vi "Main_scan.vi"() -> ()   [LabVIEW 2018]
uses:
  Positional stage/G/Control 1.ctl
  D:/Labview/examples/Instrument IO/Serial/support/Serial - Settings.ctl
  D:/Labview/examples/Instrument IO/Serial/support/Serial - XON-XOFF Characters.ctl
  D:/Labview/examples/Instrument IO/Serial/support/Serial - ASCII Characters.ctl
  <vilib>/Instr/_visa.llb/VISA Configure Serial Port (Instr).vi
  <vilib>/Utility/file.llb/Write Delimited Spreadsheet (DBL).vi
panel:
  in  "Saves per point":i32
  out "Pixel Number":dbl[](array[numeric])
  out "Wavelength":dbl[](array[numeric])
  in  "St":refnum<visa-resource-name>="COM1"
  in  "Averages":u32=1 min=1 max=60000 step=1
  in  "Integration Time":u32=50 min=50 max=60000 step=1
  out "Waveform Graph 2":dbl[](graph)
  out "I num":i32
  in  "Translation Stage":refnum<visa-resource-name>="COM1"
  out "Translation Error":bool=TRUE
  out "TS Error":bool
  in  "Filenumber":u32=1
  in  "Y Interval":dbl
  in  "X Interval":dbl
  in  "Y Scan Number":dbl
  in  "X Scan Number":dbl
  in  "Scan":bool
  out "Position":string
  in  "Command":string="0x 0y"
  in  "Connect":bool=TRUE
  in  "Move":bool
  in  "Current Position":string
  out "Array":dbl[](array[numeric])
  in  "HeadFolder":T1=path "C:/Users/xinghua/Desktop/try_step"
  out "Image array":dbl[][](array[numeric])
  # "Average"
  # "Intergration time"
  # "Spec port"
  # "Single Move"
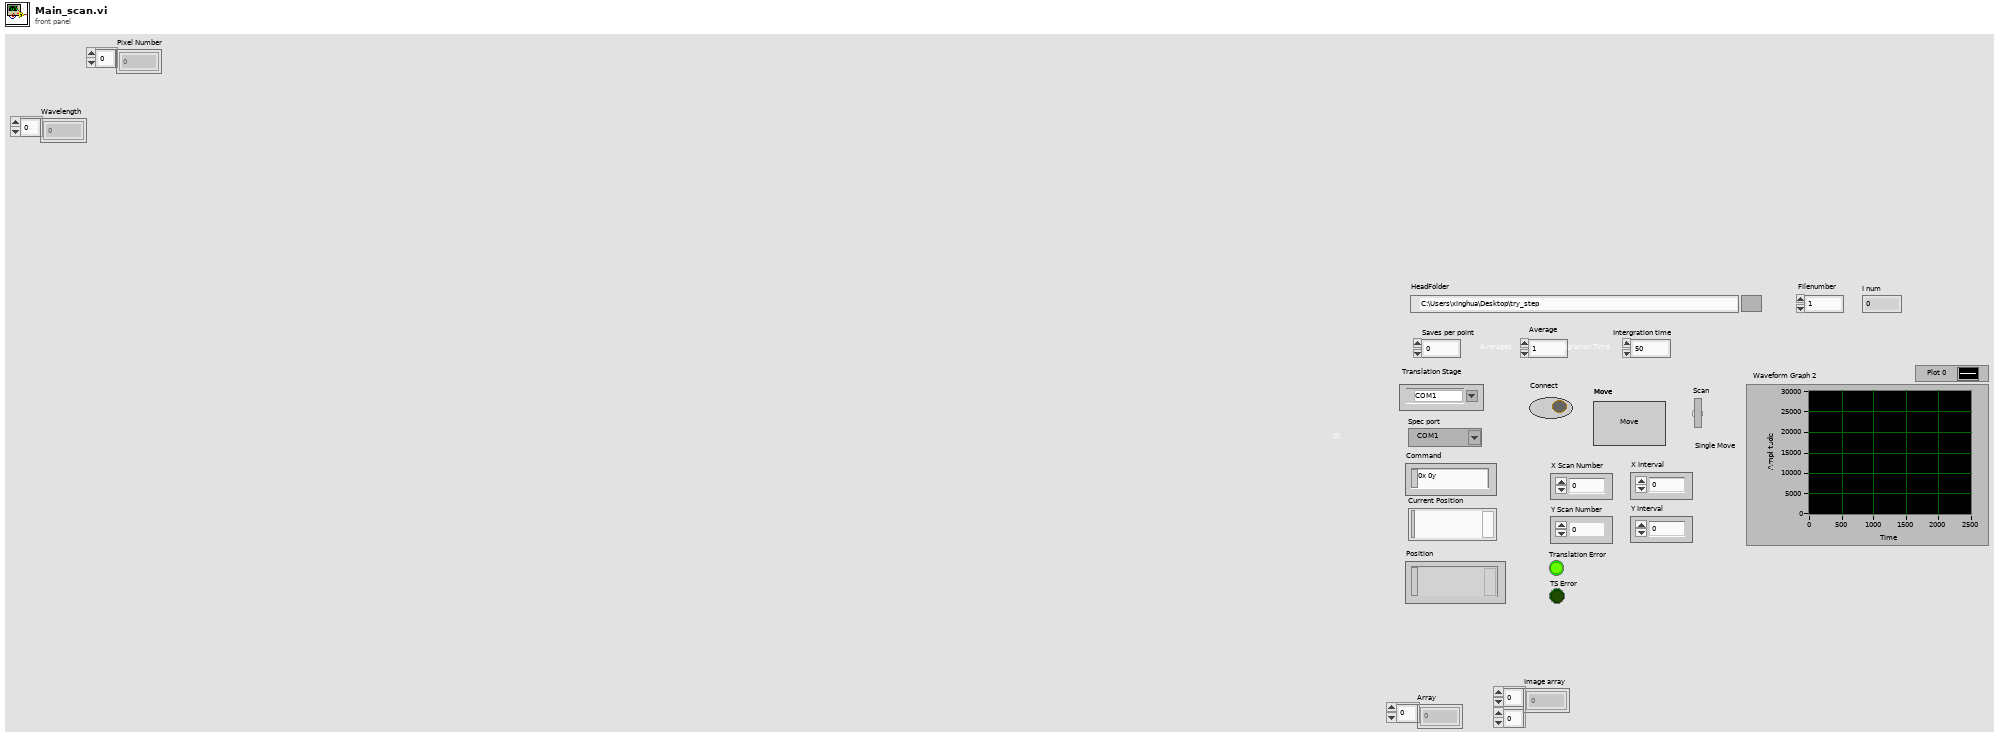
[diagram p1: front panel]
types:
  T1 = typedef "Control 1.ctl" = path
  T2 = typedef "Serial - XON-XOFF Characters.ctl" = cluster{"XON":T3, "XOFF":T3}
  T3 = typedef "Serial - ASCII Characters.ctl" = enum16{"NUL", "SOH", "STX", "ETX", "EOT", "ENQ", "ACK", "BEL", "BS", "HT", "LF", "VT", "FF", "CR", "SO", "SI", "DLE", "DC1", "DC2", "DC3", "DC4", "NAK", "SYN", "ETB", "CAN", "EM", "SUB", "ESC", "FS", "GS", "RS", "US", "SP", "!", "\"", "#", "$", "%", "&", "'", "(", ")", "*", "+", ",", "- (-)", ".", "/", "0", "1", "2", "3", "4", "5", "6", "7", "8", "9", ":", ";", "<", "=", ">", "?", "@", "A", "B", "C", "D", "E", "F", "G", "H", "I", "J", "K", "L", "M", "N", "O", "P", "Q", "R", "S", "T", "U", "V", "W", "X", "Y", "Z", "[", "\\", "]", "^", "_", "`", "a", "b", "c", "d", "e", "f", "g", "h", "i", "j", "k", "l", "m", "n", "o", "p", "q", "r", "s", "t", "u", "v", "w", "x", "y", "z", "{", "|", "}", "~"}
  T4 = typedef "Serial - Settings.ctl" = cluster{"baud rate":u32, "data bits":u16, "parity":enum16{"None", "Odd", "Even", "Mark", "Space"}, "stop bits":u16, "flow control":u16}
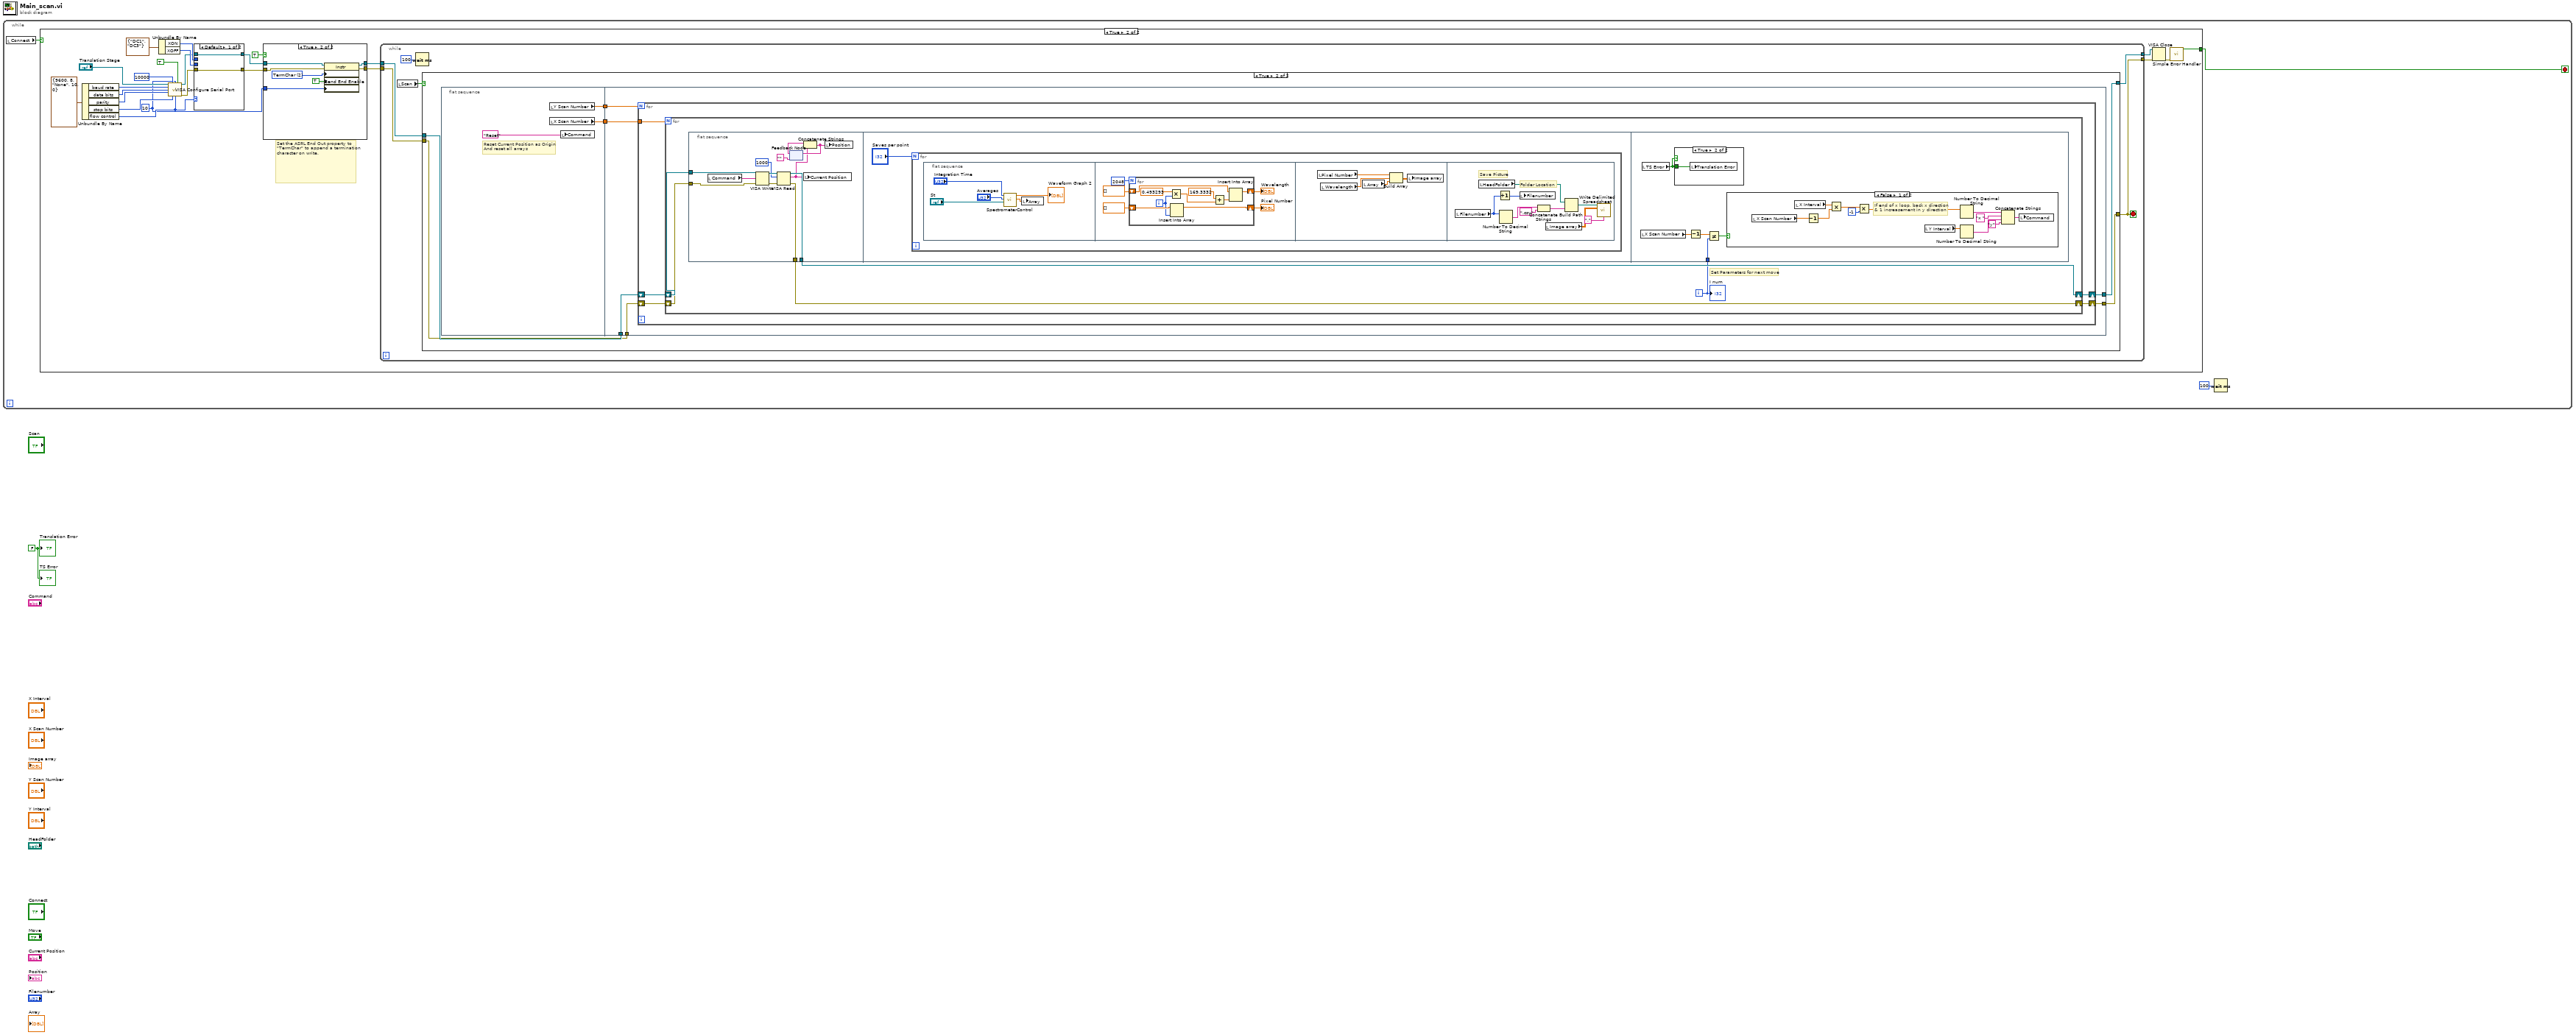
[diagram p0: block diagram]
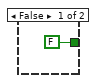
[diagram p2: hidden frame]
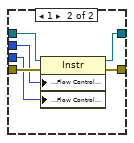
[diagram p4: hidden frame]
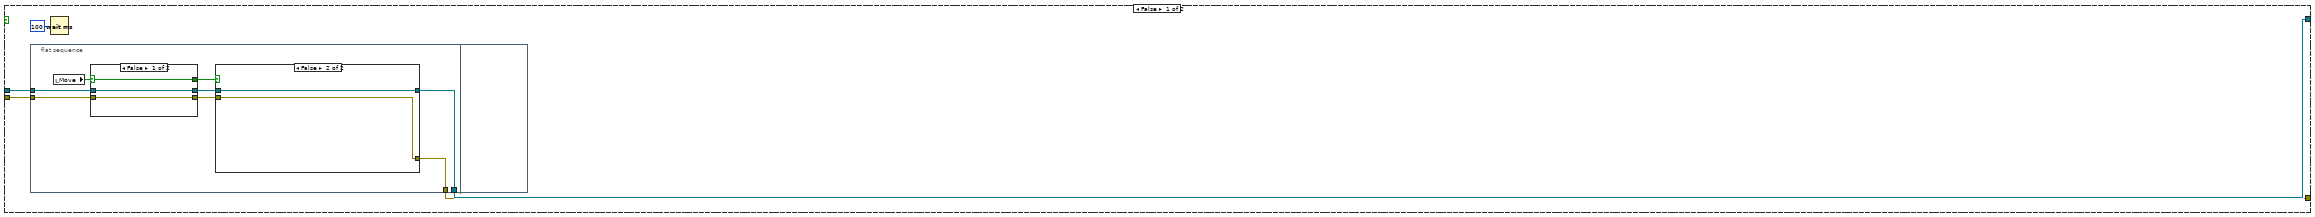
[diagram p5: hidden frame]
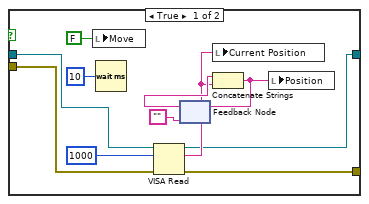
[diagram p6: hidden frame]
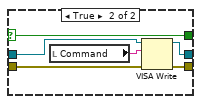
[diagram p7: hidden frame]
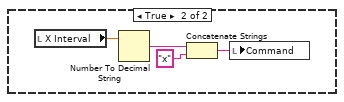
[diagram p8: hidden frame]
diagram:
  w1 = FALSE
  n1 = while {
    stop <- w2 stop-if-true
    n2 = local read "Connect"() -> (w4:bool)
    n3 = case shown="True" w4 {
      tunnel: [FALSE ("error?") w6] -> w2
      frame False {
      }
      frame True {
        w16 = u8 10 ("Termination Character")
        # "Set the ASRL End Out property to \"TermChar\" to append a termination character on write."
        n4 = Unbundle By Name(T4 {"baud rate"=9600, "data bits"=8, "parity"=enum."None", "stop bits"=10, "flow control"=0} ("input cluster")) -> ("baud rate"=w24:u32, "data bits"=w23:u16, "parity"=w22:enum16{"None", "Odd", "Even", "Mark", "Space"}, "stop bits"=w21:u16, "flow control"=w25:u16)
        n5 = Unbundle By Name(T2 {"XON"=enum."DC1", "XOFF"=enum."DC3"} ("input cluster")) -> ("XON"=w26:T3, "XOFF"=w27:T3)
        n6 = call-poly "VISA Configure Serial Port"("VISA resource name"="Translation Stage", "timeout (10sec)"=u32 10000, "termination char\n(0xA = '\\n' = LF)"=w16, "Enable Termination\nChar (T)"=TRUE ("End Read on Termination Character?"), "baud rate (9600)"=w24, "data bits (8)"=w23, "parity (0:none)"=w22, "stop bits (10: 1 bit)"=w21, "flow control (0:none)"=w25) -> ("VISA resource name out"=w20:refnum<visa-resource-name>, "error out"=w19:errorcluster)  [unwired: 1 in, 4 out]
        n7 = case shown="Default" w25 {
          tunnel: [w39 w46] -> w28
          tunnel: [w40 w45] -> w29
          tunnel: w19 -> [w39 w44]
          tunnel: w20 -> [w40 w43]
          tunnel: w26 -> [_ w42]
          tunnel: w27 -> [_ w41]
          frame Default {
          }
          frame 1 {
            n8 = property class="Instr"(reference=w43, error in=w44, "Serial Settings:Flow Control XON Character"=w42, "Serial Settings:Flow Control XOFF Character"=w41) -> (reference out=w45:refnum<visa-resource-name>, error out=w46:errorcluster)
          }
        }
        n9 = case shown="True" TRUE ("End Write on Termination Character?") {
          tunnel: w29 -> [w30 w38]
          tunnel: w28 -> [w31 w37]
          tunnel: [w30 w36] -> w11
          tunnel: [w31 w35] -> w10
          tunnel: w16 -> [_ w33]
          frame False {
          }
          frame True {
            w34 = u16 2 items=["None", "LastBit", "TermChar", "Break"] ("Serial Settings:Serial End Mode for Writes")
            n10 = property class="Instr"(reference=w38, error in=w37, "Serial Settings:End Mode for Writes"=w34, "Message Based Settings:Send End Enable"=TRUE, "Message Based Settings:Termination Character"=w33) -> (reference out=w36:refnum<visa-resource-name>, error out=w35:errorcluster)
          }
        }
        n11 = while {
          tunnel: w11 -> [w51]
          tunnel: w10 -> [w50]
          tunnel: [w47] -> w8
          tunnel: [w48] -> w7
          stop <- w47 stop-if-true
          n12 = local read "Scan"() -> (w52:bool)
          n13 = Wait (ms)(milliseconds to wait=u32 100) -> ()  [unwired: 1 out]
          n14 = case shown="True" w52 {
            tunnel: w51 -> [w57 w91]
            tunnel: w50 -> [w56 w90]
            tunnel: [w54 w89] -> w48
            tunnel: [w53 w88] -> w47
            frame False {
              n15 = flat-sequence {
                tunnel: w57 -> [w61]
                tunnel: w56 -> [w60]
                tunnel: [w59] -> w54
                tunnel: [w58] -> w53
                frame #0 {
                  n16 = local read "Move"() -> (w65:bool)
                  n17 = case shown="False" w65 {
                    selector: w65 -> [w81 w84]
                    tunnel: [w79 w87] -> w64
                    tunnel: [w80 w85] -> w63
                    tunnel: [w81 w84] -> w62
                    tunnel: w61 -> [w80 w83]
                    tunnel: w60 -> [w79 w82]
                    frame False {
                    }
                    frame True {
                      n18 = local read "Command"() -> (w86:string)
                      n19 = VISA Write(VISA resource name=w83, write buffer=w86, error in (no error)=w82) -> (VISA resource name out=w85:refnum<visa-resource-name>, error out=w87:errorcluster)  [unwired: 1 out]
                    }
                  }
                  n20 = case shown="False" w62 {
                    tunnel: w63 -> [w76 w78]
                    tunnel: w64 -> [w75 w77]
                    tunnel: [w68 w78] -> w59
                    tunnel: [w67 w77] -> w58
                    frame True {
                      n21 = local write "Move"(FALSE) -> ()
                      n22 = Wait (ms)(milliseconds to wait=u32 10) -> ()  [unwired: 1 out]
                      n23 = VISA Read(VISA resource name=w76, byte count=u32 1000 ("Read Count"), error in (no error)=w75) -> (VISA resource name out=w68:refnum<visa-resource-name>, read buffer=w70:string, error out=w67:errorcluster)  [unwired: 1 out]
                      n24 = feedback #1("") -> (w73:string)
                      n25 = local write "Current Position"(w70) -> ()
                      n26 = Concatenate Strings(w73, w70) -> (w69:string)
                      n27 = feedback-in #1(w69) -> ()
                      n28 = local write "Position"(w69) -> ()
                    }
                    frame False {
                    }
                  }
                }
                frame #1 {
                }
              }
              n29 = Wait (ms)(milliseconds to wait=u32 100) -> ()  [unwired: 1 out]
            }
            frame True {
              n30 = flat-sequence {
                tunnel: [w95] -> w93
                tunnel: [w94] -> w92
                tunnel: w93 -> [w102]
                tunnel: w92 -> [w101]
                tunnel: w91 -> [w100]
                tunnel: w90 -> [w99]
                tunnel: [w98] -> w89
                tunnel: [w97] -> w88
                frame #0 {
                  # "Reset Current Position as Origin\nAnd reset all arrays"
                  n31 = local read "Y Scan Number"() -> (w95:dbl)
                  n32 = local read "X Scan Number"() -> (w94:dbl)
                  n33 = local write "Command"("Reset") -> ()
                }
                frame #1 {
                  n34 = for {
                    N: w102 -> [_]
                    tunnel: w101 -> [w107]
                    shift-right: [w104] -> w98
                    shift-left: w100 -> [w106]
                    shift-right: [w103] -> w97
                    shift-left: w99 -> [w105]
                    n35 = for {
                      N: w107 -> [_]
                      shift-right: [w110] -> w104
                      shift-left: w106 -> [w112]
                      shift-right: [w109] -> w103
                      shift-left: w105 -> [w111]
                      i -> [w108]
                      # "Set Parameters for next move"
                      n36 = flat-sequence {
                        tunnel: w112 -> [w124]
                        tunnel: w111 -> [w123]
                        tunnel: [w122] -> w110
                        tunnel: [w121] -> w109
                        tunnel: w108 -> [w159]
                        frame #0 {
                          n37 = local read "Command"() -> (w117:string)
                          n38 = VISA Write(VISA resource name=w124, write buffer=w117, error in (no error)=w123) -> (VISA resource name out=w116:refnum<visa-resource-name>, error out=w115:errorcluster)  [unwired: 1 out]
                          n39 = VISA Read(VISA resource name=w116, byte count=u32 1000, error in (no error)=w115) -> (VISA resource name out=w122:refnum<visa-resource-name>, read buffer=w114:string, error out=w121:errorcluster)  [unwired: 1 out]
                          n40 = feedback #2("") -> (w119:string)
                          n41 = Concatenate Strings(w119, w114) -> (w118:string)
                          n42 = feedback-in #2(w118) -> ()
                          n43 = local write "Current Position"(w114) -> ()
                          n44 = local write "Position"(w118) -> ()
                        }
                        frame #1 {
                          n45 = for {
                            N: "Saves per point" -> [_]
                            n46 = flat-sequence {
                              frame #0 {
                                n47 = call "SpectrometerControl.vi"("Spectrometer Port"="St", "Averages"="Averages", "Integration Time"="Integration Time") -> ("Array"=w130:dbl[], "Waveform Graph"=→"Waveform Graph 2":dbl[])  [unwired: 6 in, 1 out]
                                n48 = local write "Array"(w130) -> ()
                              }
                              frame #1 {
                                n49 = for {
                                N: 2048 -> [_]
                                shift-right: [w143] -> w134
                                shift-left: dbl[] [] -> [w144]
                                shift-right: [w137] -> w135
                                shift-left: dbl[] [] -> [w142]
                                i -> [w136]
                                n50 = Multiply(x=0.493293, y=w136) -> (x*y=w140:dbl)
                                n51 = Insert Into Array(array=w144, new element=w136) -> (w143:dbl[])  [unwired: 1 in]
                                n52 = Add(x=169.3332, y=w140) -> (x+y=w138:dbl)
                                n53 = Insert Into Array(array=w142, new element=w138) -> (w137:dbl[])  [unwired: 1 in]
                                }
                                "Wavelength" <- w135
                                "Pixel Number" <- w134
                              }
                              frame #2 {
                                n54 = local read "Pixel Number"() -> (w147:dbl[])
                                n55 = local read "Wavelength"() -> (w148:dbl[])
                                n56 = local read "Array"() -> (w146:dbl[])
                                n57 = Build Array(w147, w148, w146) -> (w145:dbl[][])
                                n58 = local write "Image array"(w145) -> ()
                              }
                              frame #3 {
                                # "Folder Location"
                                # "Save Picture"
                                n59 = local read "Filenumber"() -> (w156:u32)
                                n60 = local read "HeadFolder"() -> (w155:T1)
                                n61 = Increment(x=w156) -> (x+1=w153:u32)
                                n62 = Number To Decimal String(number=w156) -> (decimal integer string=w154:string)  [unwired: 1 in]
                                n63 = local write "Filenumber"(w153) -> ()
                                n64 = Concatenate Strings(w154, ".csv" ("string")) -> (w157:string)
                                n65 = local read "Image array"() -> (w152:dbl[][])
                                n66 = Build Path(base path=w155, name or relative path=w157) -> (appended path=w151:path)
                                n67 = call-poly <vilib>:"Write Delimited Spreadsheet.vi"("file path (dialog if empty)"=w151, "2D data"=w152, "delimiter (\\t)"=",") -> ()  [unwired: 11 in, 2 out]
                              }
                            }
                          }
                        }
                        frame #2 {
                          n68 = local read "X Scan Number"() -> (w161:dbl)
                          n69 = local read "TS Error"() -> (w162:bool)
                          n70 = case shown="True" w162 {
                            tunnel: w162 -> [_ w179]
                            frame False {
                            }
                            frame True {
                              n71 = local write "Translation Error"(w179) -> ()
                            }
                          }
                          n72 = Decrement(x=w161) -> (x-1=w160:dbl)
                          n73 = Not Equal?(x=w160, y=w159) -> (x != y?=w158:bool)
                          n74 = case shown="False" w158 {
                            frame False {
                              # "If end of x loop, back x direction \n& 1 increasement in y direction"
                              n75 = local read "X Scan Number"() -> (w173:dbl)
                              n76 = local read "X Interval"() -> (w172:dbl)
                              n77 = Decrement(x=w173) -> (x-1=w174:dbl)
                              n78 = Multiply(x=w172, y=w174) -> (x*y=w171:dbl)
                              n79 = Multiply(x=w171, y=-1) -> (x*y=w169:dbl)
                              n80 = local read "Y Interval"() -> (w168:dbl)
                              n81 = Number To Decimal String(number=w169) -> (decimal integer string=w167:string)  [unwired: 1 in]
                              n82 = Number To Decimal String(number=w168) -> (decimal integer string=w165:string)  [unwired: 1 in]
                              n83 = Concatenate Strings(w167, "x ", w165, "y") -> (w163:string)
                              n84 = local write "Command"(w163) -> ()
                            }
                            frame True {
                              n85 = local read "X Interval"() -> (w178:dbl)
                              n86 = Number To Decimal String(number=w178) -> (decimal integer string=w177:string)  [unwired: 1 in]
                              n87 = Concatenate Strings(w177, "x") -> (w175:string)
                              n88 = local write "Command"(w175) -> ()
                            }
                          }
                        }
                      }
                      "I num" <- w108
                    }
                  }
                }
              }
            }
          }
        }
        n89 = VISA Close(VISA resource name=w7, error in (no error)=w8) -> (error out=w9:errorcluster)
        n90 = call <vilib>:"Simple Error Handler.vi"("error in (no error)"=w9) -> ("error?"=w6:bool)  [unwired: 1 in, 7 out]
      }
    }
    n91 = Wait (ms)(milliseconds to wait=u32 100) -> ()  [unwired: 1 out]
  }
  "Translation Error" <- w1
  "TS Error" <- w1
